vi "SistemaRiego.vi"() -> ()   [LabVIEW 2010]
uses:
  <vilib>/Platform/TimedLoop/XDataNode/XDataNode.xnode
  <vilib>/Platform/TimedLoop/XDataNode/timing_clust.ctl
  <vilib>/Platform/TimedLoop/XDataNode/nitl_modes.ctl
  <vilib>/Platform/TimedLoop/XDataNode/wakeup.ctl
  <vilib>/Instr/_visa.llb/VISA Configure Serial Port (Instr).vi
  <vilib>/Platform/TimedLoop/XDataNode/XDNodeRunTimeDep.lvlib
panel:
  out "x*y 2":dbl
  out "x*y":dbl
  out "Boolean 2":bool
  in  "Min Humedad (%)":u8(slide) scale=0.0..100.0
  out "Boolean":bool
  out "var t 2":i32
  out "Resistencia (ohmios)":dbl(graph)
  out "Tanque":i32(slide) scale=0.0..100.0
  out "Humedad":dynamicdata(graph)
  in  "Max Humedad (%)":u8(slide) scale=0.0..100.0
  in  "Period                :":i64=1000
  in  "Flow control    :":u16(ring) items=["None"=0, "XON/XOFF"=1, "RTS/CTS"=2, "DTR/DSR"=4]
  in  "Stop bits         :":u16(ring)=10 items=["1.0"=10, "1.5"=15, "2.0"=20]
  in  "Paridad            :":u16(ring) items=["None", "Odd", "Even", "Mark", "Space"]
  in  "Data bits          :":u16=8 min=5 max=8 step=1
  in  "VISA resource : name:":refnum<visa-resource-name>="COM1"
  in  "Baud rate         :":u32=9600
  in  "stop":bool
  out "Read buffer":string
  out "var t":i32
  # "Sistema Riego"
  # "Configuracion Serial"
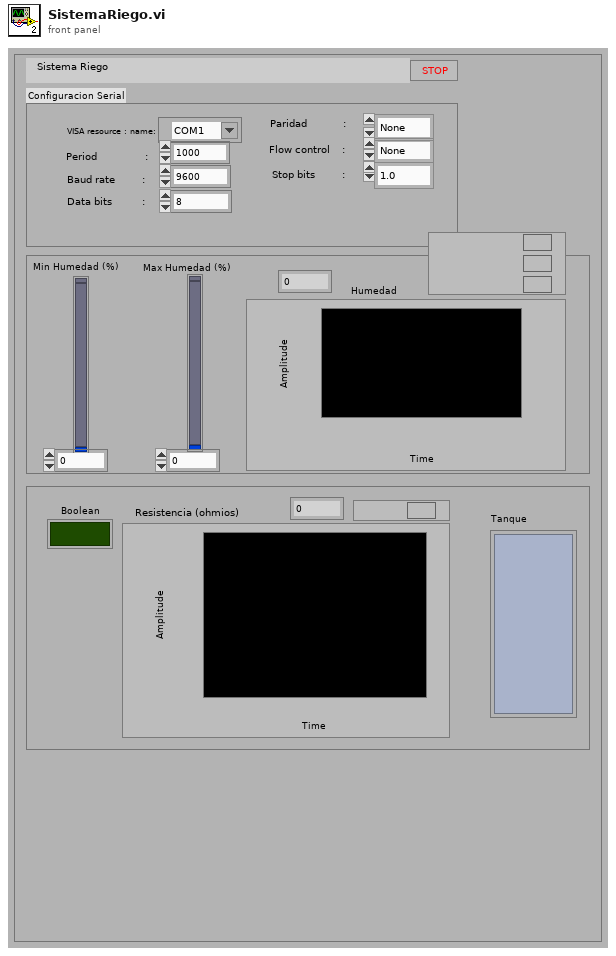
[diagram p1: front panel]
types:
  T1 = typedef "XDNodeRunTimeDep.lvlib/timing_clust.ctl" = cluster{"Expected End [f-1]":u64, "Actual End [f-1]":u64, "Finished Late? [f-1]":bool, "Expected End [i-1]":u64, "Actual End [i-1]":u64, "Finished Late? [i-1]":bool, "Expected Start [i]":u64, "Actual Start [i]":u64, "Expected Start [f]":u64, "Actual Start [f]":u64, "Source Name":string, "Structure Name":string, "Period":i64, "Deadline":i64, "Offset":i64, "Start":i64, "Priority":i32, "Timeout":i32, "Mode":T2, "Wakeup Reason":T3, "Error":errorcluster, "Source Type":string, "Secondary Source Type":string, "Global End Time":u64, "Global Start Time":u64, "Frame Duration":u64, "Iteration Duration":u64, "Assigned CPU":i32, "I/O Scan Engine Mode":u32}
  T2 = typedef "XDNodeRunTimeDep.lvlib/nitl_modes.ctl" = enum32{"No Change", "Process missed periods, maintain original phase", "Discard missed periods, maintain original phase", "Process missed periods, ignore original phase", "Discard missed periods, ignore original phase"}
  T3 = typedef "XDNodeRunTimeDep.lvlib/wakeup.ctl" = enum32{"Normal", "Aborted", "Asynchronous wakeup", "Timing source error", "Timed loop error", "Timeout"}
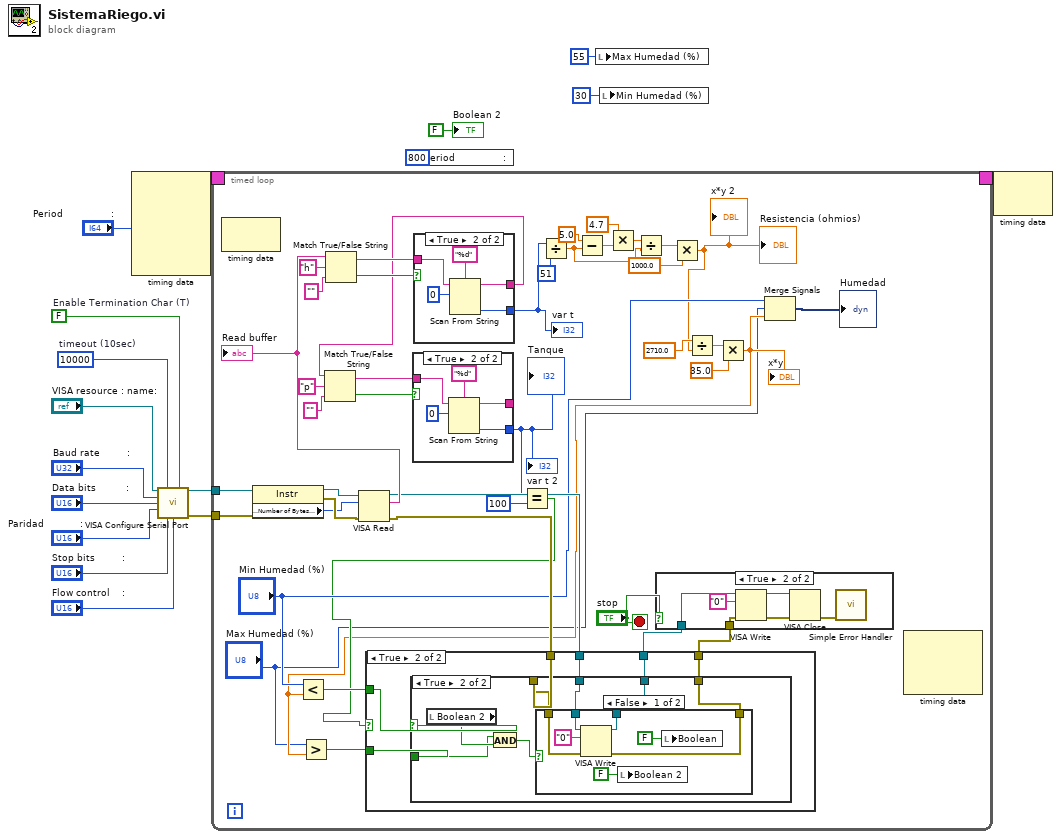
[diagram p0: block diagram]
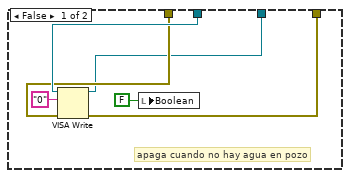
[diagram p2: hidden frame]
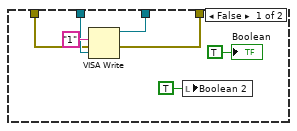
[diagram p3: hidden frame]
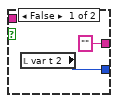
[diagram p5: hidden frame]
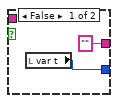
[diagram p6: hidden frame]
diagram:
  w11 = FALSE  # Enable Termination Char (T)
  w12 = u32 10000  # timeout (10sec)
  n1 = node-c288("Period                :") -> (w17:T1)  [unwired: 4 in]
  n2 = call-poly "VISA Configure Serial Port"("VISA resource name"="VISA resource : name:", "timeout (10sec)"=w12, "Enable Termination\nChar (T)"=w11, "baud rate (9600)"="Baud rate         :", "data bits (8)"="Data bits          :", "parity (0:none)"="Paridad            :", "stop bits (10: 1 bit)"="Stop bits         :", "flow control (0:none)"="Flow control    :") -> ("VISA resource name out"=w7:refnum<visa-resource-name>, "error out"=w6:errorcluster)  [unwired: 6 in]
  n3 = timed-loop {
    timing: w17 -> [_]
    timing-out: [_] -> w16
    tunnel: w7 -> [w51]
    tunnel: w6 -> [w50]
    stop <- "stop" stop-if-true
    n4 = node-c288() -> ()  [unwired: 1 in, 1 out]
    n5 = property class="Instr"(reference=w51, error in=w50) -> (reference out=w52:refnum<visa-resource-name>, error out=w59:errorcluster, "Serial Settings:Number of Bytes at Serial Port"=w58:u32)
    n6 = VISA Read(VISA resource name=w52, byte count=w58, error in (no error)=w59) -> (VISA resource name out=w49:refnum<visa-resource-name>, read buffer=w57:string, error out=w48:errorcluster)  [unwired: 1 out]
    "Read buffer" <- w57
    n7 = Match True/False String(2:"" ("false string"), 3:"h" ("true string"), 4:w57) -> (0:w55:bool, 1:w54:string)
    n8 = case shown="True" w55 {
      tunnel: w54 -> [_ w106]
      tunnel: ["" w105] -> w43
      tunnel: [w103 w104] -> w30
      frame False {
        n9 = local read "var t"() -> (w103:i32)
      }
      frame True {
        n10 = Scan From String(format string="%d", input string=w106, initial scan location=u32 0) -> (remaining string=w105:string, output 1=w104:i32)  [unwired: 2 in, 2 out]
      }
    }
    "var t" <- w30
    n11 = Match True/False String(2:"" ("false string"), 3:"p" ("true string"), 4:w43) -> (0:w45:bool, 1:w46:string)
    n12 = case shown="True" w45 {
      tunnel: w46 -> [_ w99]
      tunnel: ["" w98] -> _
      tunnel: [w96 w97] -> w38
      frame False {
        n13 = local read "var t 2"() -> (w96:i32)
      }
      frame True {
        n14 = Scan From String(format string="%d", input string=w99, initial scan location=u32 0) -> (remaining string=w98:string, output 1=w97:i32)  [unwired: 2 in, 2 out]
      }
    }
    "Tanque" <- w38
    "var t 2" <- w38
    n15 = Equal?(x=w38, y=100) -> (x = y?=w34:bool)
    n16 = Divide(x=w30, y=51) -> (x/y=w24:dbl)
    n17 = Subtract(x=5.0, y=w24) -> (x-y=w27:dbl)
    n18 = Multiply(x=4.7, y=w27) -> (x*y=w25:dbl)
    n19 = Divide(x=w25, y=w24) -> (x/y=w23:dbl)
    n20 = Multiply(x=w23, y=1000.0) -> (x*y=w18:dbl)
    "Resistencia (ohmios)" <- w18
    "x*y 2" <- w18
    n21 = Divide(x=2710.0 ("y"), y=w18) -> (x/y=w21:dbl)
    n22 = Multiply(x=w21, y=35.0) -> (x*y=w33:dbl)
    "x*y" <- w33
    n23 = Less?(x="Min Humedad (%)", y=w33) -> (x < y?=w36:bool)
    n24 = Greater?(x="Max Humedad (%)", y=w33) -> (0:w35:bool)
    n25 = case shown="True" w34 {
      tunnel: w49 -> [w63 w71]
      tunnel: w48 -> [w62 w70]
      tunnel: w35 -> [_ w69]
      tunnel: [w60 w68] -> w41
      tunnel: [w61 w67] -> w40
      tunnel: w36 -> [_ w66]
      frame False {
        # "apaga cuando no hay agua en pozo"
        n26 = VISA Write(VISA resource name=w63, write buffer="0", error in (no error)=w62) -> (VISA resource name out=w61:refnum<visa-resource-name>, error out=w60:errorcluster)  [unwired: 1 out]
        n27 = local write "Boolean"(FALSE ("Boolean")) -> ()
      }
      frame True {
        n28 = case shown="True" w66 {
          tunnel: w71 -> [w77 w85]
          tunnel: w70 -> [w74 w84]
          tunnel: [w76 w83] -> w67
          tunnel: [w75 w82] -> w68
          tunnel: w69 -> [_ w80]
          frame False {
            n29 = VISA Write(VISA resource name=w77, write buffer="1", error in (no error)=w74) -> (VISA resource name out=w76:refnum<visa-resource-name>, error out=w75:errorcluster)  [unwired: 1 out]
            n30 = local write "Boolean 2"(TRUE ("Boolean 2")) -> ()
            "Boolean" <- TRUE ("Boolean")
          }
          frame True {
            n31 = local read "Boolean 2"() -> (w81:bool)
            n32 = And(x=w80, y=w81) -> (x .and. y?=w79:bool)
            n33 = case shown="False" w79 {
              tunnel: [w91 w93] -> w83
              tunnel: [w90 w94] -> w82
              tunnel: w85 -> [w88 w93]
              tunnel: w84 -> [w87 w94]
              frame False {
                n34 = VISA Write(VISA resource name=w88, write buffer="0", error in (no error)=w87) -> (VISA resource name out=w91:refnum<visa-resource-name>, error out=w90:errorcluster)  [unwired: 1 out]
                n35 = local write "Boolean 2"(FALSE ("Boolean 2")) -> ()
                n36 = local write "Boolean"(FALSE ("Boolean")) -> ()
              }
              frame True {
              }
            }
          }
        }
      }
    }
    n37 = case shown="True" "stop" {
      tunnel: w41 -> [_ w111]
      tunnel: w40 -> [_ w110]
      frame False {
      }
      frame True {
        n38 = VISA Write(VISA resource name=w110, write buffer="0", error in (no error)=w111) -> (VISA resource name out=w113:refnum<visa-resource-name>, error out=w112:errorcluster)  [unwired: 1 out]
        n39 = VISA Close(VISA resource name=w113, error in (no error)=w112) -> (error out=w114:errorcluster)
        n40 = call <vilib>:"Simple Error Handler.vi"("error in (no error)"=w114) -> ()  [unwired: 4 in, 5 out]
      }
    }
    n41 = Merge Signals("Min Humedad (%)", "Max Humedad (%)", w33) -> (→"Humedad":dynamicdata)
    n42 = node-c288() -> ()  [unwired: 3 in, 1 out]
  }
  n43 = local write "Period                :"(i64 800 ("Period")) -> ()
  n44 = local write "Max Humedad (%)"(u8 55 ("Max Humedad (%)")) -> ()
  n45 = local write "Min Humedad (%)"(u8 30 ("Min Humedad (%)")) -> ()
  n46 = node-c288(w16) -> ()  [unwired: 1 out]
  "Boolean 2" <- FALSE ("Boolean 2")
